vi "wrap.StackState.vi"(0 "class.GLue in":refnum<class "class.GLue.lvclass">, 11 "error in (no error)":errorcluster) -> (4 "class.GLue out":refnum<class "class.GLue.lvclass">, 8 "TopType":T1, 13 "Size":i32, 15 "error out":errorcluster)   [LabVIEW 2014, in "GLue.lvlib" / "class.GLue.lvclass"]
uses:
  class.GLue.lvclass
  typedef.Types.ctl
  class.GLue.lvclass/class.GLue.ctl
  Resources/GLue.dll
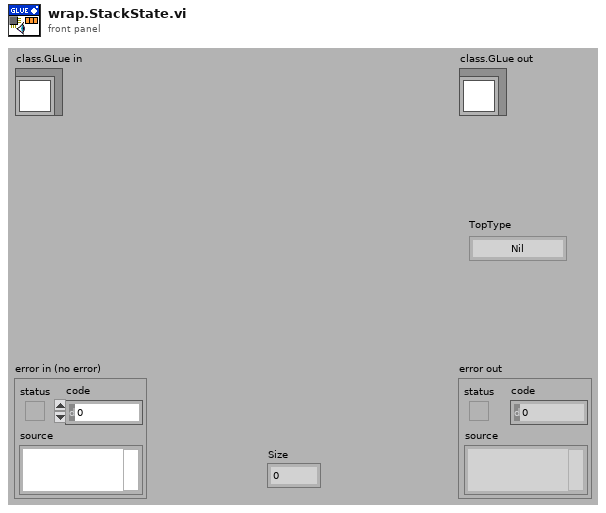
[diagram p1: front panel]
types:
  T1 = typedef "GLue.lvlib/class.GLue.lvclass/typedef.Types.ctl" = enum16{"Nil", "Bool", "LightUserData", "Number", "String", "Table", "Function", "UserData", "Thread"}
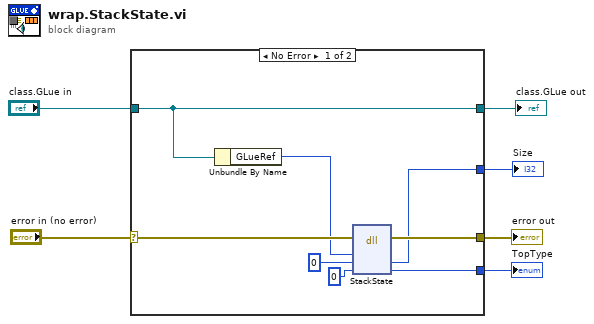
[diagram p0: block diagram]
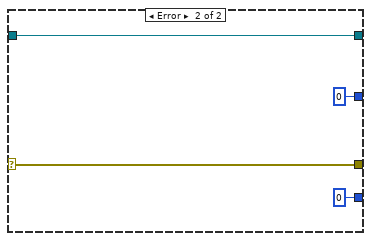
[diagram p2: hidden frame]
diagram:
  n1 = case shown="No Error" "error in (no error)" {
    selector: "error in (no error)" -> [w13 w18]
    tunnel: [w12 w18] -> w5
    tunnel: [w14 w17] -> w3
    tunnel: "class.GLue in" -> [w14 w17]
    tunnel: [w10 0 ("Size")] -> w2
    tunnel: [w9 0 ("TopType")] -> w1
    frame No Error {
      n2 = Unbundle By Name(w14) -> ("GLueRef"=w11:i64)
      n3 = dll-call lib="C:/Users/Antonie/Documents/work/glue/trunk/Resources/GLue.dll" fn="StackState"(error in=w13, "GLue"=w11, "Size"=0, "TopType"=0 ("Bool")) -> (error out=w12:errorcluster, "Size"=w10:i32, "TopType"=w9:i32)  [unwired: 4 in, 1 out]
    }
    frame Error {
    }
  }
  "error out" <- w5
  "class.GLue out" <- w3
  "Size" <- w2
  "TopType" <- w1
